vi "initialize.vi"(0 "HGF_ThreadTask":refnum<class "HGF_ThreadTask.lvclass">, 3 "initializationData":variant, 5 "error in (no error)":errorcluster, 7 "binaryString":string, 8 "I8 Array":i8[](array[numeric]), 9 "prependSize? (T)":bool, 11 "byteOrder (0:big-endian, network order)":T1(ring)) -> (14 "dup HGF_ThreadTask":refnum<class "HGF_ThreadTask.lvclass">, 17 "found?":bool, 19 "error out":errorcluster)   [LabVIEW 2014, in "HGF_BaseClasses.lvlib" / "HGF_ThreadTask.lvclass"]
doc: "This is a dynamic dispatch VI to be implemented by child classes to initialize their attributes.\n\n<B>Recommendation:</B> Use Variant for initialization data."
uses:
  HGF_ThreadTask.lvclass
  HGF_Event/HGF_Event.lvclass
  HGF_Base/HGF_Base.lvclass
  HGF_TriggeredEvent/HGF_TriggeredEvent.lvclass
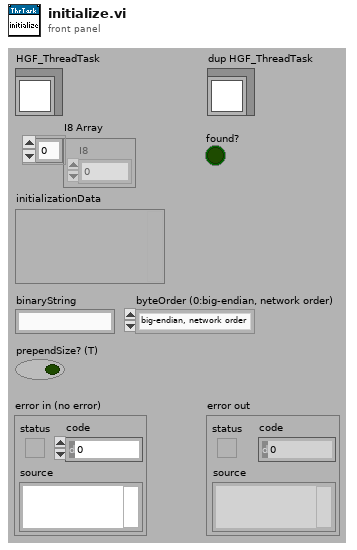
[diagram p1: front panel]
types:
  T1 = enum16{"big-endian, network order", "native, host order", "little-endian"}
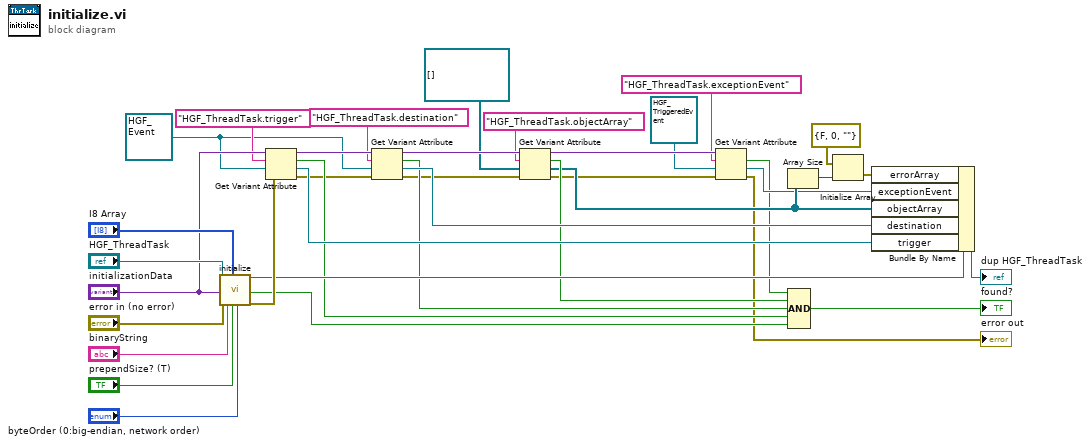
[diagram p0: block diagram]
diagram:
  w24 = refnum<class "HGF_Event.lvclass"> refnum ("HGF_BaseClasses.lvlib:HGF_Event.lvclass")
  n1 = call-parent "initialize.vi"("HGF_Base"="HGF_ThreadTask", "initializationData"="initializationData", "error in (no error)"="error in (no error)", "binaryString"="binaryString", "I8 Array"="I8 Array", "prependSize? (T)"="prependSize? (T)", "byteOrder (0:big-endian, network order)"="byteOrder (0:big-endian, network order)") -> ("dup HGF_Base"=w30:refnum<class "HGF_ThreadTask.lvclass">, "found?"=w28:bool, "error out"=w31:errorcluster)  [unwired: 1 in, 9 out]
  n2 = Get Variant Attribute(Variant="initializationData", name="HGF_ThreadTask.trigger", default value (empty Variant)=w24, error in=w31) -> (duplicate Variant=w26:variant, found=w29:bool, value=w32:refnum<class "HGF_Event.lvclass">, error out=w25:errorcluster)
  n3 = Get Variant Attribute(Variant=w26, name="HGF_ThreadTask.destination", default value (empty Variant)=w24, error in=w25) -> (duplicate Variant=w19:variant, found=w22:bool, value=w23:refnum<class "HGF_Event.lvclass">, error out=w16:errorcluster)
  n4 = Get Variant Attribute(Variant=w19, name="HGF_ThreadTask.objectArray", default value (empty Variant)=refnum<class>[] [] ("objectArray"), error in=w16) -> (duplicate Variant=w7:variant, found=w17:bool, value=w15:refnum<class>[], error out=w3:errorcluster)
  n5 = Get Variant Attribute(Variant=w7, name="HGF_ThreadTask.exceptionEvent", default value (empty Variant)=refnum<class "HGF_TriggeredEvent.lvclass"> refnum ("exceptionEvent"), error in=w3) -> (found=w1:bool, value=w4:refnum<class "HGF_TriggeredEvent.lvclass">, error out=→"error out":errorcluster)  [unwired: 1 out]
  n6 = Array Size(array=w15) -> (size(s)=w14:i32)
  n7 = Compound Arithmetic op=AND(w1, w17, w22, w29, w28) -> (→"found?":bool)
  n8 = Initialize Array(errorcluster {"status"=FALSE, "code"=0, "source"=""} ("error out"), w14) -> (w12:errorcluster[])
  n9 = Bundle By Name(cluster=w30, "errorArray"=w12, "exceptionEvent"=w4, "objectArray"=w15, "destination"=w23, "trigger"=w32) -> (→"dup HGF_ThreadTask":refnum<class "HGF_ThreadTask.lvclass">)
